vi "test_client.vi"() -> ()   [LabVIEW 2017, in "server.lvlib"]
uses:
  server.lvlib
panel:
  in  "data in":string
  in  "stop":bool
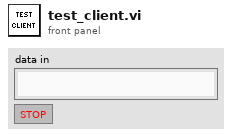
[diagram p1: front panel]
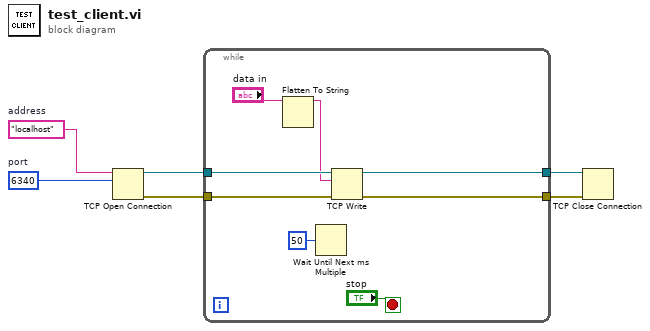
[diagram p0: block diagram]
diagram:
  w5 = u16 6340  # port
  w6 = "localhost"  # address
  n1 = TCP Open Connection(address=w6, remote port or service name=w5) -> (connection ID=w3:refnum<k5>, error out=w4:errorcluster)  [unwired: 3 in]
  n2 = while {
    tunnel: w4 -> [w13]
    tunnel: w3 -> [w12]
    tunnel: [w11] -> w2
    tunnel: [w10] -> w1
    stop <- "stop" stop-if-true
    n3 = Flatten To String(anything="data in") -> (data string=w7:string)  [unwired: 3 in, 2 out]
    n4 = Wait Until Next ms Multiple(millisecond multiple=u32 50) -> ()  [unwired: 1 out]
    n5 = TCP Write(connection ID=w12, data in=w7, error in (no error)=w13) -> (connection ID out=w10:refnum<k5>, error out=w11:errorcluster)  [unwired: 1 in, 1 out]
  }
  n6 = TCP Close Connection(connection ID=w1, error in (no error)=w2) -> ()  [unwired: 1 in, 2 out]
